vi "TIFF_4_Write_To_New_File.vi"(8 "error in (no error)":errorcluster, 9 "Input cluster":T1, 11 "Destination Image Path":path=path "C:/Users/Sebastien/Desktop/TIFF/data_000000_Metadata.tif") -> (0 "Error Out":errorcluster, 1 "output cluster":T1)   [LabVIEW 2025]
doc: "This software was created to prototype writing metadata to a TIFF file with a single image.\n\n<B>Usage:</B> This software is free to use, copy or plagiariaze. It is provided \"as-is\", and no technical support will be provided. The copyright is retained by NASA Marshall Space Flight Center.\n\n<B>Testing:</B> This software was tested by A) verifying that operations were completed successfully using LabVIEW 2009 on Windows XP, .NET version 4.0 and B) Windows Vista Microsoft Office Picture Manager was able to read and display the output file and C) Windows Vista Windows Photo Gallery was able to read and display the output file and the Description and D) Adobe Photoshop for Macintosh was able to correctly load and display the image and all the metadata.\n\n<B>Note:</B> This software requires .NET version 4.0\n\n<B>Warning:</B> This software will overwrite the destination file if it exists.\n\nThis software originally developed by:\nDerek Mayer\nBAE Systems - Technology Solutions & Services\n308 Voyager Way\nHuntsville, AL 35806\n(256) 890-8000\nwww.mevatec.com\nwww.baesystems.com/TSS\nSeptember 2010"
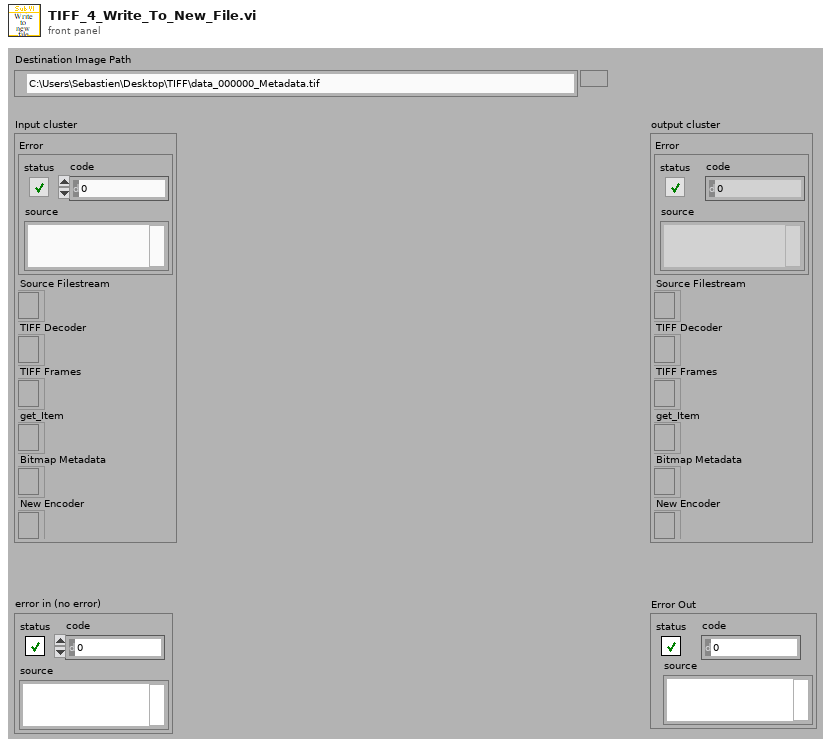
[diagram p1: front panel]
types:
  T1 = cluster{"Error":errorcluster, "Source Filestream":refnum<k24>, "TIFF Decoder":refnum<k24>, "TIFF Frames":refnum<k24>, "get_Item":refnum<k24>, "Bitmap Metadata":refnum<k24>, "New Encoder":refnum<k24>}
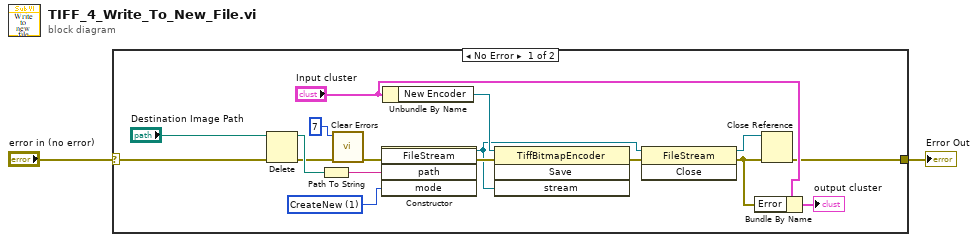
[diagram p0: block diagram]
diagram:
  n1 = case shown="No Error" "error in (no error)" {
    selector: "error in (no error)" -> [w7 w20]
    tunnel: [w3 w20] -> w2
    frame No Error {
      w16 = 1 items=["CreateNew"=1, "Create"=2, "Open"=3, "OpenOrCreate"=4, "Truncate"=5, "Append"=6] ("mode")
      n2 = Delete(path (use dialog)="Destination Image Path", error in=w7) -> (deleted path=w18:path, error out=w6:errorcluster)  [unwired: 3 in, 1 out]
      n3 = Path To String(path=w18) -> (string=w17:string)
      n4 = call <vilib>:"Clear Errors.vi"("error in (no error)"=w6, "specific error code to clear (0: all)"=7) -> ("error out"=w5:errorcluster)  [unwired: 4 in, 1 out]
      n5 = constructor class="FileStream"(error in=w5, "path"=w17, "mode"=w16) -> (reference out=w13:refnum<k24>, error out=w14:errorcluster)  [unwired: 2 in, 3 out]
      n6 = Unbundle By Name("Input cluster") -> ("New Encoder"=w15:refnum<k24>)
      n7 = invoke class="TiffBitmapEncoder" method="Save"(reference=w15, error in=w14, "stream"=w13) -> (error out=w12:errorcluster)  [unwired: 1 in, 3 out]
      n8 = invoke class="FileStream" method="Close"(reference=w13, error in=w12) -> (reference out=w11:refnum<k24>, error out=w8:errorcluster)  [unwired: 1 in, 1 out]
      n9 = Bundle By Name(cluster="Input cluster", "Error"=w8) -> (→"output cluster":T1)
      n10 = Close Reference(reference=w11, error in (no error)=w8) -> (error out=w3:errorcluster)
    }
    frame Error {
    }
  }
  "Error Out" <- w2
